vi "SaveDataPathBuilder.vi"(10 "DataTypeSuffix":string, 11 "Inst name":string) -> (3 "Path name Out":path)   [LabVIEW 2014]
uses:
  Globals/Meas_global.vi
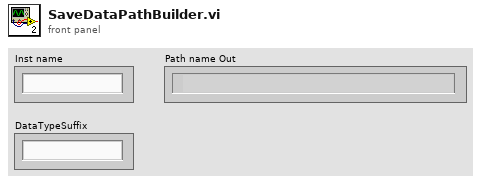
[diagram p1: front panel]
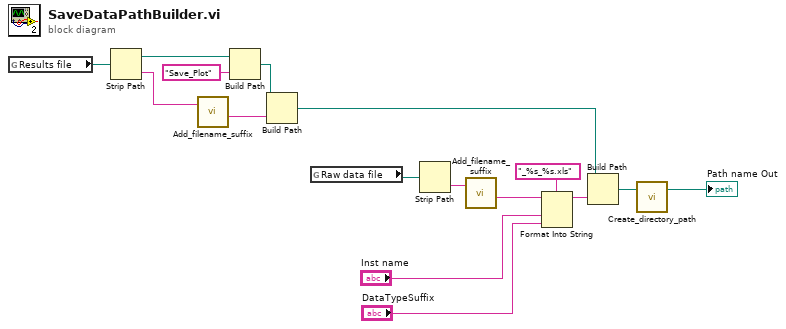
[diagram p0: block diagram]
diagram:
  n1 = global read "Meas_global.vi" "Results file"() -> (w1:path)
  n2 = Strip Path(path=w1) -> (stripped path=w4:path, name=w2:string)
  n3 = call "Add_filename_suffix.vi"("Filename"=w2) -> ("Base name"=w3:string)  [unwired: 1 in, 3 out]
  n4 = Build Path(base path=w4, name or relative path="Save_Plot") -> (appended path=w6:path)
  n5 = Build Path(base path=w6, name or relative path=w3) -> (appended path=w12:path)
  n6 = global read "Meas_global.vi" "Raw data file"() -> (w9:path)
  n7 = Strip Path(path=w9) -> (name=w7:string)  [unwired: 1 out]
  n8 = call "Add_filename_suffix.vi"("Filename"=w7) -> ("Base name"=w10:string)  [unwired: 1 in, 3 out]
  n9 = Format Into String(format string="_%s_%s.xls", initial string=w10, "Inst name", "DataTypeSuffix") -> (resulting string=w11:string)  [unwired: 1 in, 1 out]
  n10 = Build Path(base path=w12, name or relative path=w11) -> (appended path=w15:path)
  n11 = call "Create_directory_path.vi"("Path name"=w15) -> ("Path name Out"=→"Path name Out":path)  [unwired: 1 in, 1 out]
